vi "Divide.vi"(1 "A":T1={"Array Num"=[1, 2, 3], "Decimal Index"=0, "stop"=FALSE}, 2 "B":T1={"Array Num"=[1, 2, 3], "Decimal Index"=0, "stop"=FALSE}, 4 "digits":i32=10) -> (5 "A/B":T1={"Array Num"=[1, 2, 3], "Decimal Index"=0, "stop"=FALSE})   [LabVIEW 2025]
uses:
  Number.ctl
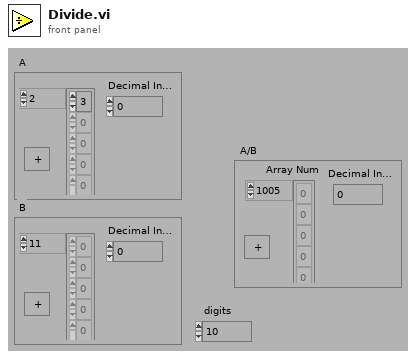
[diagram p1: front panel]
types:
  T1 = typedef "Number.ctl" = cluster{"Array Num":i8[], "Decimal Index":i32, "stop":bool}
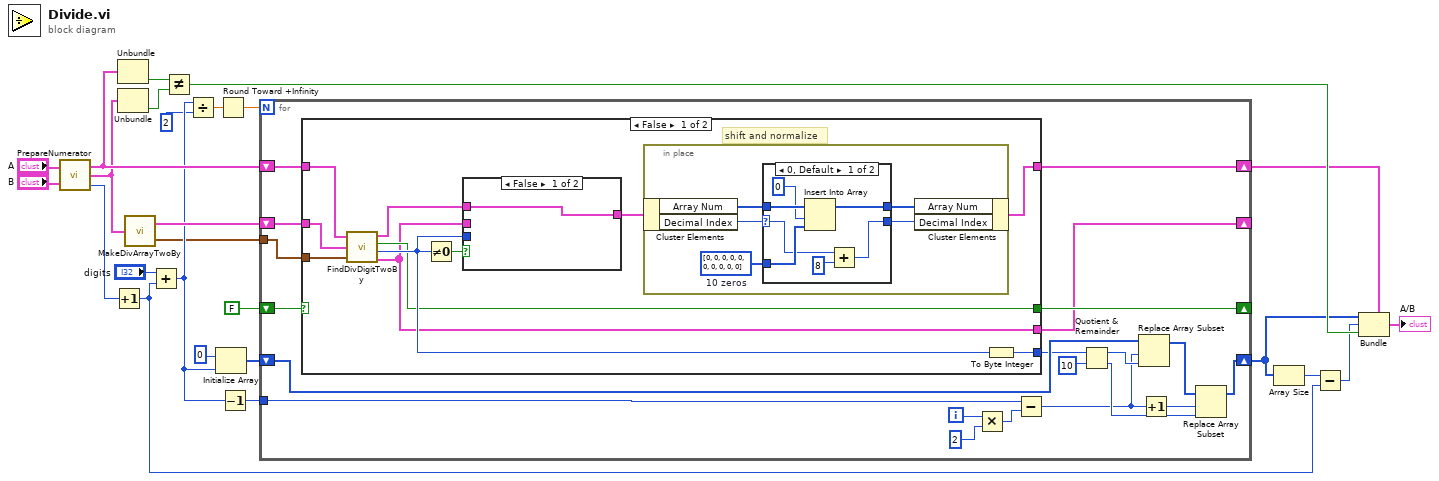
[diagram p0: block diagram]
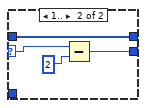
[diagram p2: hidden frame]
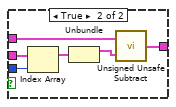
[diagram p3: hidden frame]
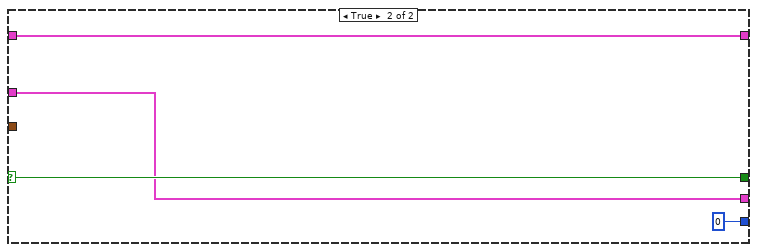
[diagram p4: hidden frame]
diagram:
  n1 = call "PrepareNumerator.vi"("A"="A", "B"="B") -> ("Normalized A"=w15:T1, "B copy"=w14:T1, "Shifted"=w13:i32)
  n2 = Increment(x=w13) -> (x+1=w8:i32)
  n3 = Unbundle(w15) -> ("stop"=w7:bool)  [unwired: 2 out]
  n4 = Unbundle(w14) -> ("stop"=w23:bool)  [unwired: 2 out]
  n5 = call "MakeDivArrayTwoBy.vi"("B"=w14) -> ("output array"=w6:cluster{"A":T1, "stop":bool}[], "Denom Info"=w1:cluster{"Denom":i32, "Offset":i32})
  n6 = Add(x="digits", y=w8) -> (x+y=w4:i32)
  n7 = Not Equal?(x=w7, y=w23) -> (x != y?=w22:bool)
  n8 = Divide(x=w4, y=i8 2) -> (x/y=w5:dbl)
  n9 = Initialize Array(i8 0, w4) -> (w11:i8[])
  n10 = Round Toward +Infinity(x=w5) -> (ceil(x): smallest int >= x=w2:dbl)
  n11 = Decrement(x=w4) -> (x-1=w12:i32)
  n12 = for {
    N: w2 -> [_]
    shift-right: [w45] -> w21
    shift-left: w15 -> [w44]
    shift-right: [w42] -> _
    shift-left: FALSE -> [w43]
    shift-right: [w41] -> w9
    shift-left: w11 -> [w36]
    tunnel: w12 -> [w40]
    shift-right: [w39] -> _
    shift-left: w6 -> [w38]
    tunnel: w1 -> [w26]
    i -> [w31]
    n13 = case shown="False" w43 {
      selector: w43 -> [_ w81]
      tunnel: [w51 w83] -> w45
      tunnel: [w56 i8 0] -> w33
      tunnel: w44 -> [w50 w83]
      tunnel: w38 -> [w48 w80]
      tunnel: [w53 w81] -> w42
      tunnel: [w47 w80] -> w39
      tunnel: w26 -> [w46 _]
      frame False {
        # "shift and normalize"
        n14 = call "FindDivDigitTwoBy.vi"("Normalized A"=w50, "premultiplied array"=w48, "Denom Info"=w46) -> ("A Copy"=w49:T1, "Exact Divide"=w53:bool, "Digit"=w55:i32, "premultiplied array out"=w47:cluster{"A":T1, "stop":bool}[])
        n15 = Not Equal To 0?(x=w55) -> (x != 0?=w54:bool)
        n16 = case shown="False" w54 {
          tunnel: [w73 w78] -> w52
          tunnel: w49 -> [w73 w79]
          tunnel: w47 -> [_ w77]
          tunnel: w55 -> [_ w76]
          frame False {
          }
          frame True {
            n17 = Index Array(array=w77, index=w76) -> (element=w75:cluster{"A":T1, "stop":bool})
            n18 = Unbundle(w75) -> ("A"=w74:T1)  [unwired: 1 out]
            n19 = call "Unsigned Unsafe Subtract.vi"("B"=w74, "A"=w79) -> ("A-B"=w78:T1)
          }
        }
        n20 = in-place {
          w61 = i8[] [0, 0, 0, 0, 0, 0, 0, 0, 0, 0]  # 10 zeros
          n21 = in-place-cluster #1(w52) -> ("Array Num"=w58:i8[], "Decimal Index"=w57:i32)
          n22 = case shown="0, Default" w57 {
            selector: w57 -> [w65 w70]
            tunnel: [w64 w72] -> w59
            tunnel: w58 -> [w68 w71]
            tunnel: [w67 w71] -> w60
            tunnel: w61 -> [w66 _]
            frame 0, Default {
              n23 = Insert Into Array(array=w68, index=0, new element=w66) -> (w67:i8[])
              n24 = Add(x=w65, y=8) -> (x+y=w64:i32)
            }
            frame 1.. {
              n25 = Subtract(x=w70, y=2) -> (x-y=w72:i32)
            }
          }
          n26 = in-place-cluster #1("Array Num"=w60, "Decimal Index"=w59) -> (w51:T1)
        }
        n27 = To Byte Integer(number=w55) -> (8bit integer=w56:i8)
      }
      frame True {
      }
    }
    n28 = Multiply(x=w31, y=2) -> (x*y=w29:i32)
    n29 = Subtract(x=w40, y=w29) -> (x-y=w28:i32)
    n30 = Quotient & Remainder(x=w33, y=10) -> (x-y*floor(x/y)=w35:i32, floor(x/y)=w34:i32)
    n31 = Replace Array Subset(array=w36, new element=w35, index=w28) -> (w32:i8[])
    n32 = Increment(x=w28) -> (x+1=w27:i32)
    n33 = Replace Array Subset(array=w32, new element=w34, index=w27) -> (w41:i8[])
  }
  n34 = Array Size(array=w9) -> (size(s)=w20:i32)
  n35 = Subtract(x=w20, y=w8) -> (x-y=w19:i32)
  n36 = Bundle(cluster=w21, "Array Num"=w9, "Decimal Index"=w19, "stop"=w22) -> (→"A/B":T1)
